vi "ExMovCollect.vi"() -> ()   [LabVIEW 2010]
panel:
  out "Current Wavelength":string
  in  "Increment Wavelength":dbl=50.0 format="%.2f"
  in  "End Wavelength":dbl=700.0 format="%.2f"
  in  "Start Wavelength":dbl format="%.2f"
  in  "Grating Speed":dbl=2000.0 min=1.0 step=1.0 format="%.2f"
  in  "Grating number":i16=1 min=1 max=100 step=1
  out "Strip":sgl[](graph)
  in  "Temperature":dbl=-10.0 format="%.2f"
  in  "Exposure":dbl min=0.0 step=0.001 format="%.3f"
  in  "stop":bool
  out "error out":errorcluster
  in  "error in (no error)":errorcluster
  # "ExMovCollect.vi\n(Normal Spectrograph via USB/COM port)\nCamera and Spectrometer control.  This vi will open both the camera and spectrograph.  It will then move the grating to the Start Wavelength.  Data will then be collected and displayed.  The sequence will be repeated after moving the grating by the Increment Wavelength until the End Wavelength is reached.  At that time, data collection will continue until the STOP button is hit."
  # "NOTES:\nA properly configured spectometer .ini must be present in the LabVIEW folder for spectrograph operation.\n\nConsult the Toolkit documentation for more information on how to configure this file."
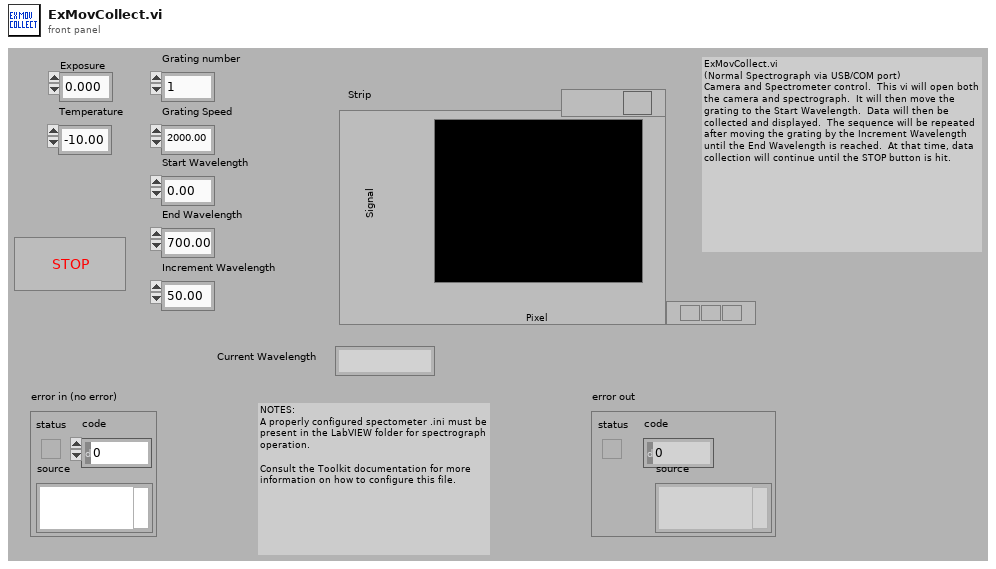
[diagram p1: front panel]
types:
  T1 = cluster{"Camera Handle":u32, "Pulser Handle":u32, "File Handle":u32, "Display Handle":u32, "Image Handle":u32}
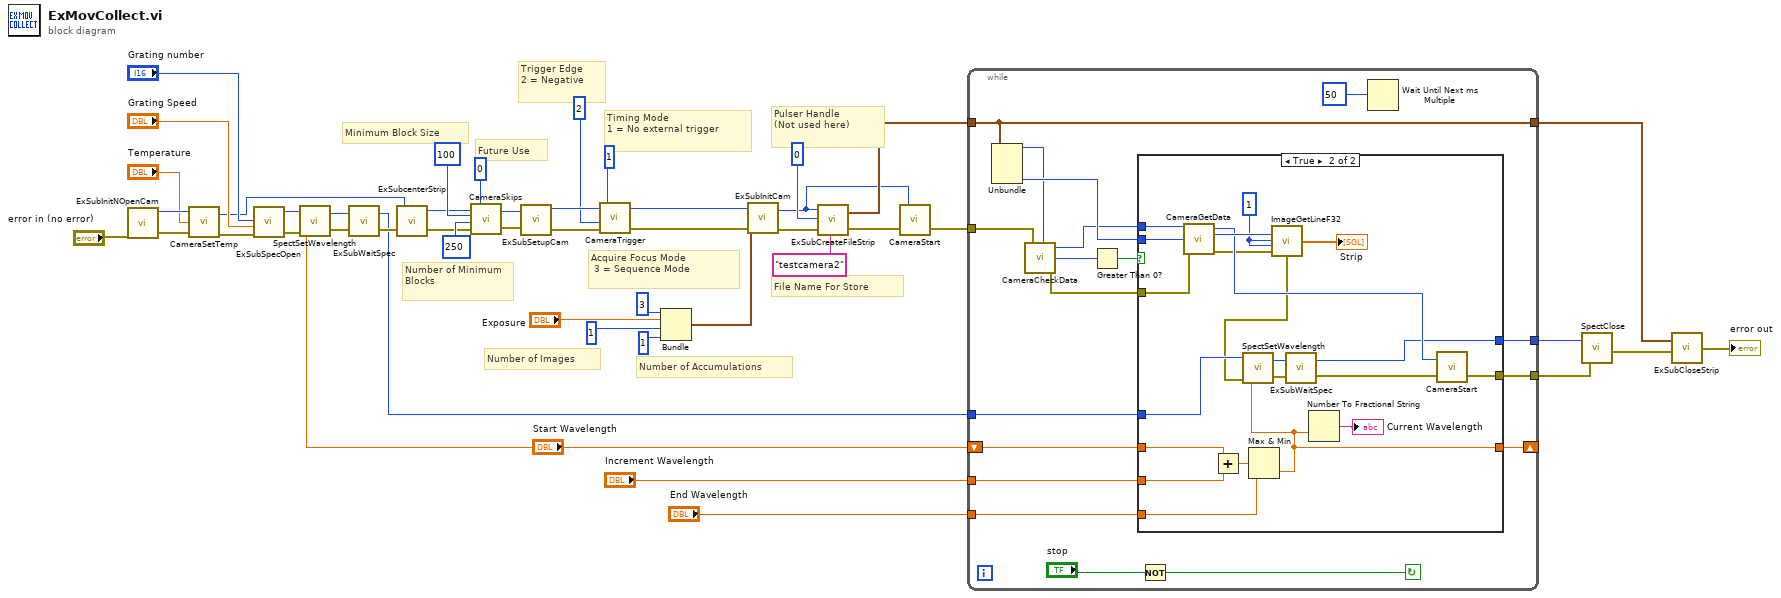
[diagram p0: block diagram]
diagram:
  # "Pulser Handle\n(Not used here)"
  # "Trigger Edge\n2 = Negative"
  # "Timing Mode\n1 = No external trigger"
  # "Future Use"
  # "Number of Minimum Blocks"
  # "Minimum Block Size"
  # "Number of Images"
  # "Number of Accumulations"
  # "Acquire Focus Mode\n 3 = Sequence Mode"
  # "File Name For Store"
  n1 = call "ExSubInitNOpenCam.vi"("error in (no error)"="error in (no error)") -> ("Camera Handle"=w2:u32, "error out"=w3:errorcluster)
  n2 = call <userlib>:"CameraSetTemp.vi"("error in (no error)"=w3, "Temperature"="Temperature", "Camera Handle"=w2) -> ("error out"=w4:errorcluster, "Camera Handle"=w5:u32)
  n3 = call "ExSubSpecOpen.vi"("error in (no error)"=w4, "Grating speed"="Grating Speed", "Grating number"="Grating number") -> ("error out"=w12:errorcluster, "Spectrometer Handle"=w6:u32)  [unwired: 1 in, 1 out]
  n4 = call <userlib>:"SpectSetWavelength.vi"("error in"=w12, "Wavelength"="Start Wavelength", "Spectrometer Handle"=w6) -> ("error out"=w17:errorcluster, "Spectrumeter Handle"=w15:u32)
  n5 = call "ExSubWaitSpec.vi"("error in (no error)"=w17, "Spectrometer Handle"=w15) -> ("error out"=w16:errorcluster, "Spectrometer handle"=w14:u32)
  n6 = call "ExSubcenterStrip.vi"("error in (no error)"=w16, "Camera Handle"=w5) -> ("error out"=w20:errorcluster, "Camera Handle"=w21:u32)
  n7 = call <userlib>:"CameraSkips.vi"("Camera Handle"=w21, "Minimum Block Size"=100, "Number of Minimum blocks"=250, "error in"=w20, "Type of Skips"=0) -> ("Camera Handle"=w24:u32, "error out"=w23:errorcluster)
  n8 = call "ExSubSetupCam.vi"("error in (no error)"=w23, "Camera Handle"=w24) -> ("error out"=w29:errorcluster, "Camera Handle"=w33:u32)
  n9 = call <userlib>:"CameraTrigger.vi"("error in"=w29, "Trigger Edge"=2, "Timing Mode"=1, "Camera Handle"=w33) -> ("error out"=w34:errorcluster, "Camera Handle"=w32:u32)
  n10 = Bundle(3, "Exposure"="Exposure", 1, 1) -> (w41:cluster{i32, "Exposure":dbl, i32, i32})  [unwired: 1 in]
  n11 = call "ExSubInitCam.vi"("error in (no error)"=w34, "Camera Information"=w41, "Camera Handle"=w32) -> ("error out"=w40:errorcluster, "Camera Handle"=w37:u32)
  n12 = call "ExSubCreateFileStrip.vi"("error in (no error)"=w40, "File and Display Name"="testcamera2", "Pulser Handle"=0, "Camera Handle"=w37) -> ("error out"=w22:errorcluster, "Handles Out"=w38:T1)
  n13 = call <userlib>:"CameraStart.vi"("error in"=w22, "Camera Handle"=w37) -> ("error out"=w25:errorcluster)  [unwired: 1 out]
  n14 = while {
    tunnel: w38 -> [w62]
    tunnel: w25 -> [w61]
    tunnel: [w59] -> w7
    tunnel: [w62] -> w36
    tunnel: w14 -> [w53]
    tunnel: "Increment Wavelength" -> [w52]
    tunnel: "End Wavelength" -> [w51]
    shift-right: [w49] -> _
    shift-left: "Start Wavelength" -> [w50]
    tunnel: [w48] -> w8
    stop <- w63 continue-if-true
    n15 = Unbundle(w62) -> ("Camera Handle"=w57:u32, "Image Handle"=w58:u32)  [unwired: 3 out]
    n16 = call <userlib>:"CameraCheckData.vi"("Camera Handle"=w57, "error in"=w61) -> ("Camera Handle"=w56:u32, "Number Of Frames Available"=w54:i32, "error out"=w60:errorcluster)
    n17 = Greater Than 0?(x=w54) -> (x > 0?=w55:bool)
    n18 = case shown="True" w55 {
      tunnel: w60 -> [w68 w88]
      tunnel: [w68 w76] -> w59
      tunnel: w58 -> [_ w85]
      tunnel: w56 -> [_ w84]
      tunnel: w53 -> [w66 w80]
      tunnel: w52 -> [_ w73]
      tunnel: w51 -> [_ w79]
      tunnel: w50 -> [w67 w72]
      tunnel: [w67 w71] -> w49
      tunnel: [w66 w70] -> w48
      frame False {
      }
      frame True {
        w86 = 1
        n19 = call <userlib>:"CameraGetData.vi"("error in"=w88, "Data Handle"=w85, "Camera Handle"=w84) -> ("error out"=w77:errorcluster, "Data Handle"=w87:u32, "Camera Handle"=w83:u32)
        n20 = Add(x=w72, y=w73) -> (x+y=w78:dbl)
        n21 = Max & Min(x=w78, y=w79) -> (min(x,y)=w71:dbl)  [unwired: 1 out]
        n22 = call <userlib>:"ImageGetLineF32.vi"("error in"=w77, "Z Position"=w86, "Y Position"=w86, "Data Handle"=w87) -> ("error out"=w74:errorcluster, "Array F32"=→"Strip":sgl[])  [unwired: 1 out]
        n23 = call <userlib>:"SpectSetWavelength.vi"("error in"=w74, "Wavelength"=w71, "Spectrometer Handle"=w80) -> ("error out"=w82:errorcluster, "Spectrumeter Handle"=w81:u32)
        n24 = call "ExSubWaitSpec.vi"("error in (no error)"=w82, "Spectrometer Handle"=w81) -> ("error out"=w69:errorcluster, "Spectrometer handle"=w70:u32)
        n25 = Number To Fractional String(number=w71) -> (F-format string=→"Current Wavelength":string)  [unwired: 3 in]
        n26 = call <userlib>:"CameraStart.vi"("error in"=w69, "Camera Handle"=w83) -> ("error out"=w76:errorcluster)  [unwired: 1 out]
      }
    }
    n27 = Not(x="stop") -> (.not. x?=w63:bool)
    n28 = Wait Until Next ms Multiple(millisecond multiple=50) -> ()  [unwired: 1 out]
  }
  n29 = call <userlib>:"SpectClose.vi"("error in"=w7, "Spectrometer Handle"=w8) -> ("error out"=w9:errorcluster)
  n30 = call "ExSubCloseStrip.vi"("error in (no error)"=w9, "Handles In"=w36) -> ("error out"=→"error out":errorcluster)
